vi "29_Sum using Shift Register and Feedback node.vi"() -> ()   [LabVIEW 2018]
panel:
  out "Sum with feed back node=":dbl
  out "Sum with shift register=":dbl
  # "Develop a HMI to find sum of the first 5 natural numbers"
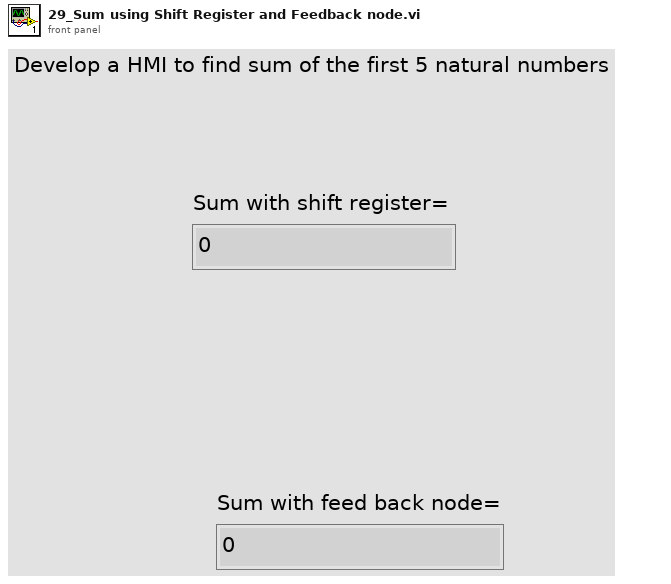
[diagram p1: front panel]
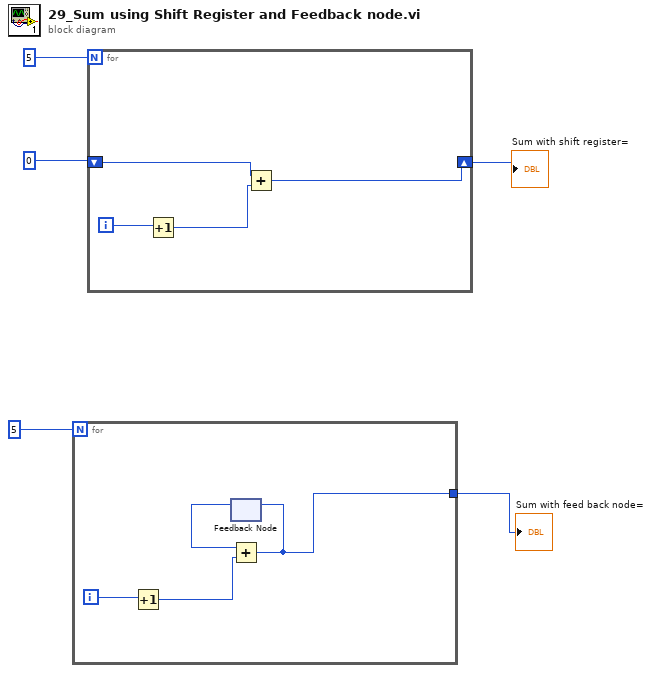
[diagram p0: block diagram]
diagram:
  n1 = for {
    N: 5 -> [_]
    tunnel: [w7] -> w1
    i -> [w9]
    n2 = Increment(x=w9) -> (x+1=w8:i32)
    n3 = feedback #1() -> (w6:i32)  [unwired: 1 in]
    n4 = Add(x=w6, y=w8) -> (x+y=w7:i32)
    n5 = feedback-in #1(w7) -> ()
  }
  "Sum with feed back node=" <- w1
  n6 = for {
    N: 5 -> [_]
    shift-right: [w12] -> w3
    shift-left: 0 -> [w13]
    i -> [w11]
    n7 = Increment(x=w11) -> (x+1=w10:i32)
    n8 = Add(x=w13, y=w10) -> (x+y=w12:i32)
  }
  "Sum with shift register=" <- w3
